vi "DrawTopics.vi"(2 "Selection":i32) -> (3 "new picture":picture, 4 "Status":string, 5 "Servers":string[](array[string]), 6 "Boundaries":cluster{i32, i32}[](array[cluster])=[{10, 22}, {30, 42}, {50, 62}])   [LabVIEW 2010]
uses:
  <vilib>/Utility/miscctls.llb/LVRectTypeDef.ctl
  MyState.ctl
panel:
  out "Status":T1[](array[typedef])
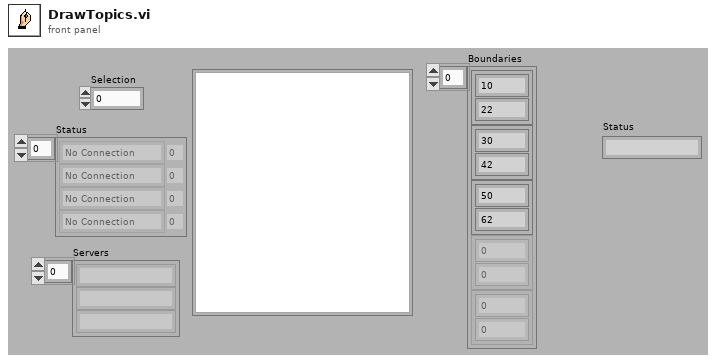
[diagram p1: front panel]
types:
  T1 = typedef "MyState.ctl" = enum16{"No Connection", "Registered", "Connected", "Close"}
  T2 = enum16{"Add Server", "Clear Server", "Clear All", "Get Info", "GetPanelInfo"}
  T3 = cluster{"left":i16, "top":i16, "right":i16, "bottom":i16}
  T4 = typedef "LVRectTypeDef.ctl" = cluster{"Left":i16, "Top":i16, "Right":i16, "Bottom":i16}
  T5 = typedef "imagedata.ctl" = cluster{"image type":i32, "image depth":i32, "image":u8[], "mask":u8[], "colors":u32[], "Rectangle":cluster{"left":i16, "top":i16, "right":i16, "bottom":i16}}
  T6 = cluster{"horizontal":enum16{"left", "center", "right"}, "vertical":enum16{"top", "center", "bottom"}}
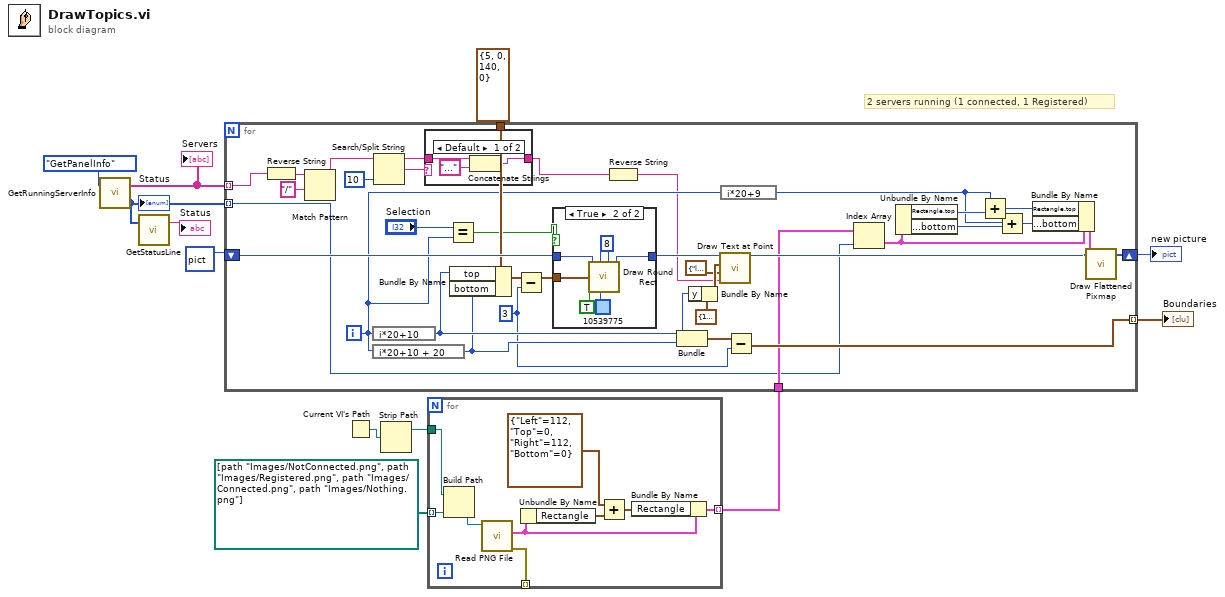
[diagram p0: block diagram]
diagram:
  # "2 servers running (1 connected, 1 Registered)"
  n1 = call "GetRunningServerInfo.vi"("Task"=T2."GetPanelInfo") -> ("Status"=w3:T1[], "Topics"=w4:string[])  [unwired: 1 in, 1 out]
  "Servers" <- w4
  "Status" <- w3
  n2 = call "GetStatusLine.vi"("Status"=w3) -> ("Status"=→"Status":string)  [unwired: 2 in]
  n3 = Current VI's Path() -> (path=w7:path)
  n4 = Strip Path(path=w7) -> (stripped path=w6:path)  [unwired: 1 out]
  n5 = for {
    tunnel: [w19] -> w8 mode=indexing
    tunnel: w6 -> [w16]
    tunnel: path[] [path "Images/NotConnected.png", path "Images/Registered.png", path "Images/Connected.png", path "Images/Nothing.png"] -> [w15] mode=indexing
    tunnel: [w13] -> _ mode=indexing
    n6 = Build Path(base path=w16, name or relative path=w15) -> (appended path=w14:path)
    n7 = call <vilib>:"Read PNG File.vi"("path to PNG file"=w14) -> ("error out"=w13:errorcluster, "image data"=w20:T5)  [unwired: 8 in, 1 out]
    n8 = Unbundle By Name(w20) -> ("Rectangle"=w18:T3)
    n9 = Add(x=T4 {"Left"=112, "Top"=0, "Right"=112, "Bottom"=0} ("Bounds"), y=w18) -> (x+y=w17:T4)
    n10 = Bundle By Name(cluster=w20, "Rectangle"=w17) -> (w19:T5)
  }
  n11 = for {
    tunnel: w4 -> [w30] mode=indexing
    shift-right: [w42] -> w12
    shift-left: picture data[5B] ("new picture") -> [w53]
    tunnel: [w48] -> w10 mode=indexing
    tunnel: T3 {"left"=5, "top"=0, "right"=140, "bottom"=0} ("rect") -> [w49]
    tunnel: w8 -> [w40]
    tunnel: w3 -> [w31] mode=indexing
    i -> [w35]
    w45 = i16 3 ("oval width")
    n12 = Reverse String(1:w30) -> (0:w29:string)
    n13 = Match Pattern(string=w29, regular expression="/") -> (before substring=w26:string)  [unwired: 1 in, 3 out]
    n14 = expression code="i*20+10"(w35) -> (w51:i32)
    n15 = expression code="i*20+10 + 20"(w35) -> (w50:i32)
    n16 = Search/Split String(string=w26, offset (0)=10) -> (substring before match=w22:string, match + rest of string=w24:string)  [unwired: 1 in, 1 out]
    n17 = case shown="Default" w24 {
      tunnel: [w60 w61] -> w23
      tunnel: w22 -> [w59 w61]
      frame Default {
        n18 = Concatenate Strings(w59, "..." ("string")) -> (w60:string)
      }
      frame "" {
      }
    }
    n19 = Equal?(x="Selection", y=w35) -> (x = y?=w43:bool)
    n20 = Bundle By Name(cluster=w49, "top"=w51, "bottom"=w50) -> (w47:T3)
    n21 = Subtract(x=w47, y=w45) -> (x-y=w46:T3)
    n22 = case shown="True" w43 {
      tunnel: w53 -> [w62 w65]
      tunnel: [w62 w64] -> w52
      tunnel: w46 -> [_ w63]
      frame False {
      }
      frame True {
        w66 = i16 8 ("oval width")
        n23 = call <vilib>:"Draw Round Rect.vi"("picture"=w65, "oval width"=w66, "rect"=w63, "fill?(F)"=TRUE, "color(black)"=u32 10539775, "oval height"=w66) -> ("new picture"=w64:picture)  [unwired: 3 in]
      }
    }
    n24 = Reverse String(1:w23) -> (0:w27:string)
    n25 = Bundle(w51, w50) -> (w55:cluster{i32, i32})  [unwired: 1 in]
    n26 = Bundle By Name(cluster=cluster{"x":i16, "y":i16} {"x"=10, "y"=0} ("origin"), "y"=w51) -> (w56:cluster{"x":i16, "y":i16})
    n27 = call <vilib>:"Draw Text at Point.vi"("text"=w27, "alignment(left, top)"=T6 {"horizontal"=enum."left", "vertical"=enum."top"}, "origin"=w56, "picture"=w52) -> ("new picture"=w41:picture)  [unwired: 6 in, 1 out]
    n28 = expression code="i*20+9"(w35) -> (w33:i32)
    n29 = Subtract(x=w55, y=w45) -> (x-y=w48:cluster{i32, i32})
    n30 = Index Array(array=w40, index=w31) -> (element=w36:T5)
    n31 = Unbundle By Name(w36) -> ("Rectangle.top"=w38:i16, "Rectangle.bottom"=w34:i16)
    n32 = Add(x=w33, y=w38) -> (x+y=w39:i32)
    n33 = Add(x=w34, y=w33) -> (x+y=w32:i32)
    n34 = Bundle By Name(cluster=w36, "Rectangle.top"=w39, "Rectangle.bottom"=w32) -> (w37:T5)
    n35 = call <vilib>:"Draw Flattened Pixmap.vi"("image data"=w37, "picture"=w41) -> ("new picture"=w42:picture)  [unwired: 7 in]
  }
  "new picture" <- w12
  "Boundaries" <- w10
